vi "Data Encapsulation Example.vi"() -> ()   [LabVIEW 2020]
doc: "This example demonstrates data encapsulation using LabVIEW object-oriented programming.\n\nEncapsulation allows you to create modular code that you can easily update or change without affecting other sections of the application. \n\nRefer to the LabVIEW Help for more information about LabVIEW object-oriented programming."
uses:
  Test Results/Test Results.lvclass
panel:
  out "error out":errorcluster
  # "This example demonstrates data encapsulation using LabVIEW object-oriented programming.\n\n\"Data encapsulation\", sometimes referred to as data hiding, is the mechanism whereby the \nimplementation details of a class are kept hidden from the user.\nThe advantage of using data encapsulation comes when the implementation of the class \nchanges but the interface remains the same.\n\nData Encapsulation allows you to create modular code that you can easily update or change \nwithout affecting other sections of the application. \n\nThis VI uses the class \"Test Results\" and initializes the test status to Failure and then \ndisplays the results of the test using a method of the class 'Display.vi'. \nNote: - This test is hard coded to fail.\n\nTo illustrate the concept of Data Encapsulation, please follow the following instructions: -\n1. Run this VI, a message box will pop up saying that the \"Test Failed. Failure time: ...\"\n2. Go-to the Project explorer and open \"Test Results.ctl\" under \"Test Results.lvclass\" \n    (The Class data is stored here).\n3. Replace the boolean control \"result\" with Numeric. Save the changes and close.\n4. Open the method \"Initialize.vi\" under \"Test Results.lvclass\" and replace the boolean control  \n     \"result\" with a Numeric control. \n5. Open the VI \"Run Test For Data Encapsulation Example.vi\" and replace the boolean 'result' \n     indicator with a Numeric. Replace the boolean constant wired to the indicator to Numeric \n     constant and set '0'.\n6. You could also optionally change the message in the method \"Display.vi\" based on the result.\n7. Save all the changes.\n8. You will be able to run this example without making any changes to the top-level VI. ( Thus \n     experiencing the power of \"Data Encapsulation\" where the change in implementation does \n     not warrant any change in the interface)\n\nRefer to the LabVIEW Help for more information about LabVIEW object-oriented programming."
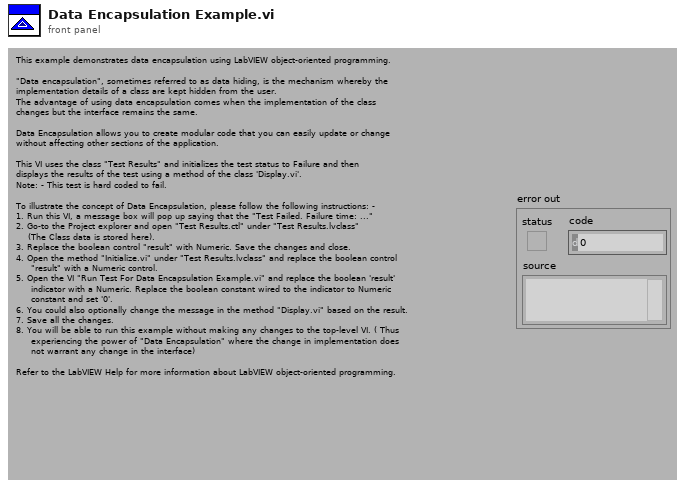
[diagram p1: front panel]
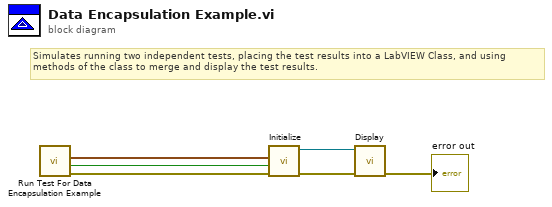
[diagram p0: block diagram]
diagram:
  # "Simulates running two independent tests, placing the test results into a LabVIEW Class, and using\nmethods of the class to merge and display the test results."
  n1 = call "Run Test For Data Encapsulation Example.vi"() -> ("error out"=w2:errorcluster, "result"=w4:bool, "time"=w5:timestamp)  [unwired: 9 in]
  n2 = call "Initialize.vi"("error in"=w2, "result"=w4, "time/date"=w5) -> ("error out"=w1:errorcluster, "test results out"=w3:refnum<class "Test Results.lvclass">)  [unwired: 7 in]
  n3 = call "Display.vi"("error in"=w1, "test results in"=w3) -> ("error out"=→"error out":errorcluster)  [unwired: 9 in]
